vi "onAddKeyValuePair.vi"(8 "error in (no error)":errorcluster, 9 "value":variant, 10 "key":string, 11 "Leaf.Properties in":refnum<class "Leaf.Properties.lvclass">) -> (0 "error out":errorcluster, 3 "Leaf.Properties out":refnum<class "Leaf.Properties.lvclass">)   [LabVIEW 2021, in "Banana.Caraya.lvlib" / "Leaf.Properties.lvclass"]
uses:
  Leaf.Properties.lvclass
  Leaf.Properties.lvclass/Leaf.Properties.ctl
  <vilib>/addons/_JKI Toolkits/Caraya/classes/Properties/Properties.lvclass
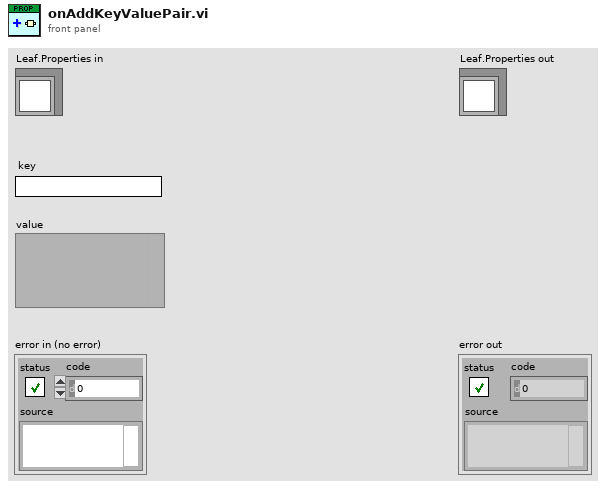
[diagram p1: front panel]
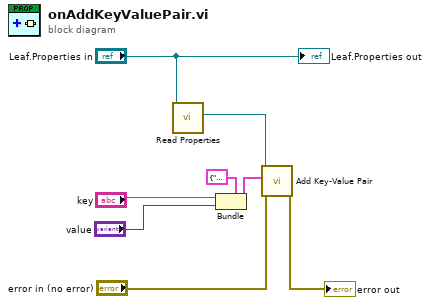
[diagram p0: block diagram]
diagram:
  n1 = call "Read Properties.vi"("Leaf.Properties in"="Leaf.Properties in") -> ("Properties"=w3:refnum<class "Properties.lvclass">)  [unwired: 9 in, 1 out]
  n2 = Bundle(cluster=cluster{"key":string, "value":variant} {"key"="", "value"=variant} ("entry"), "key"="key", "value"="value") -> (w7:cluster{"key":string, "value":variant})
  n3 = call <vilib>:"Add Key-Value Pair.vi"("error in (no error)"="error in (no error)", "entry"=w7, "Properties in"=w3) -> ("error out"=→"error out":errorcluster)  [unwired: 7 in, 1 out]
  "Leaf.Properties out" <- "Leaf.Properties in"
